vi "Flankenerkennung.vi"(10 "Eingang":bool) -> (0 "Fallende Flanke":bool, 2 "Steigende Flanke":bool)   [LabVIEW 2020, in "Allgemein.lvlib"]
uses:
  Allgemein.lvlib
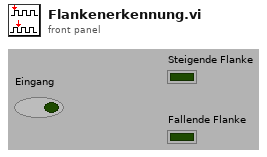
[diagram p1: front panel]
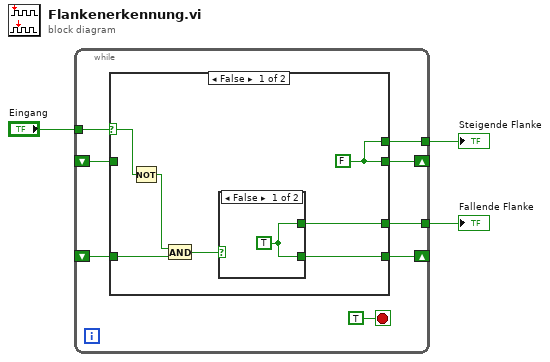
[diagram p0: block diagram]
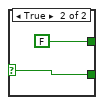
[diagram p2: hidden frame]
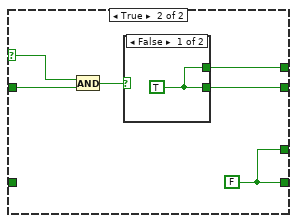
[diagram p3: hidden frame]
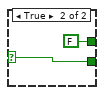
[diagram p4: hidden frame]
diagram:
  n1 = while {
    shift-right: [w10] -> _
    shift-left: _ -> [w11]
    shift-right: [w8] -> _
    shift-left: _ -> [w7]
    tunnel: "Eingang" -> [w6]
    tunnel: [w5] -> w2
    tunnel: [w4] -> w1
    stop <- TRUE stop-if-true
    n2 = case shown="False" w6 {
      selector: w6 -> [w13 w24]
      tunnel: w11 -> [_ w27]
      tunnel: [w18 w25] -> w10
      tunnel: [w18 w23] -> w5
      tunnel: [w17 w22] -> w8
      tunnel: w7 -> [w12 _]
      tunnel: [w15 w22] -> w4
      frame False {
        w18 = FALSE
        n3 = Not(x=w13) -> (.not. x?=w14:bool)
        n4 = And(x=w14, y=w12) -> (x .and. y?=w16:bool)
        n5 = case shown="False" w16 {
          selector: w16 -> [_ w20]
          tunnel: [w19 w20] -> w17
          tunnel: [w19 FALSE] -> w15
          frame False {
            w19 = TRUE
          }
          frame True {
          }
        }
      }
      frame True {
        w22 = FALSE
        n6 = And(x=w24, y=w27) -> (x .and. y?=w26:bool)
        n7 = case shown="False" w26 {
          selector: w26 -> [_ w30]
          tunnel: [w28 w30] -> w25
          tunnel: [w28 FALSE] -> w23
          frame False {
            w28 = TRUE
          }
          frame True {
          }
        }
      }
    }
  }
  "Steigende Flanke" <- w2
  "Fallende Flanke" <- w1
